vi "Get SGL Image Pixel Values.vi"(8 "error in (no error)":errorcluster, 10 "Point Array":cluster{"Numeric":i32, "Numeric":i32}[](array[cluster]), 11 "Image Refnum in":T1) -> (0 "error out":errorcluster, 2 "Pixel Values":sgl[](array[numeric]), 3 "Image Refnum out":T1)   [LabVIEW 2021, in "Image.lvlib"]
uses:
  Image.lvlib
  <vilib>/vision/Image Controls.llb/IMAQ Image.ctl
  <vilib>/vision/NI_Vision_Development_Module.lvlib
  Utilities/Utilities.lvlib
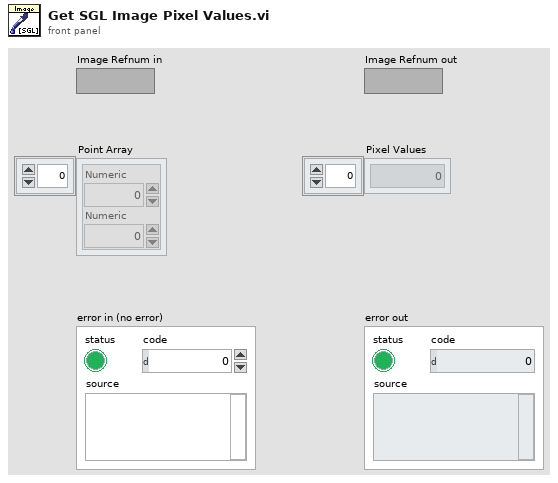
[diagram p1: front panel]
types:
  T1 = typedef "IMAQ Image.ctl" = refnum<image>
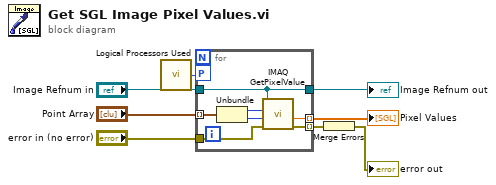
[diagram p0: block diagram]
diagram:
  n1 = call "Logical Processors Used.vi"() -> ("# Logical Processor Used"=w1:i32)  [unwired: 6 in]
  n2 = for {
    tunnel: "Point Array" -> [w11] mode=indexing
    tunnel: "Image Refnum in" -> [w9]
    tunnel: "error in (no error)" -> [w13]
    workers-P: w1 -> [_]
    tunnel: [w12] -> w4 mode=indexing
    tunnel: [w10] -> w7 mode=indexing
    tunnel: [w9] -> w3
    n3 = Unbundle(w11) -> ("Numeric"=w15:i32, "Numeric"=w14:i32)
    n4 = call "IMAQ GetPixelValue"("Image"=w9, "X Coordinate"=w15, "Y Coordinate"=w14, "error in (no error)"=w13) -> ("Pixel Value (Float)"=w12:sgl, "error out"=w10:errorcluster)  [unwired: 2 in, 3 out]
  }
  "Pixel Values" <- w4
  "Image Refnum out" <- w3
  n5 = Merge Errors(w7) -> (→"error out":errorcluster)
